vi "testAbbrevDetectorName.vi"(8 "error in (no error)":errorcluster) -> (0 "error out":errorcluster)   [LabVIEW 2016]
doc: "Test to transform the canonical detector name to the abbreviated one."
uses:
  <vilib>/addons/_JKI Toolkits/Caraya/classes/Assert/Assert.lvclass
  <vilib>/addons/_JKI Toolkits/Caraya/classes/Test/Test.lvclass
  MatOper/MatOper.lvclass
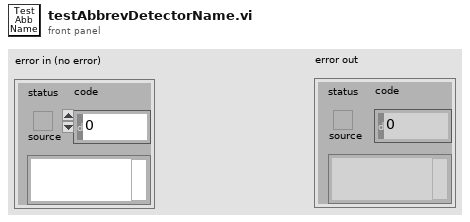
[diagram p1: front panel]
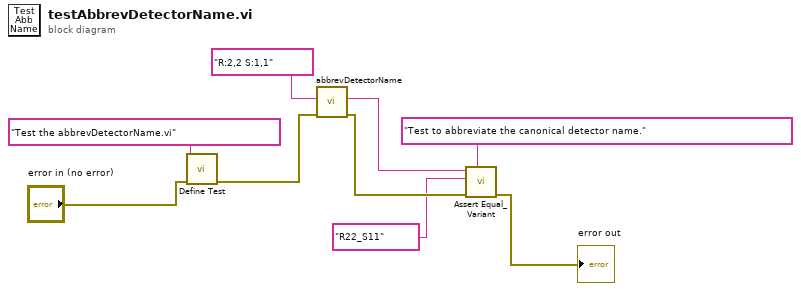
[diagram p0: block diagram]
diagram:
  n1 = call <vilib>:"Define Test.vi"("error in (no error)"="error in (no error)", "Label (VI Title)"="Test the abbrevDetectorName.vi") -> ("error out"=w5:errorcluster)  [unwired: 9 in]
  n2 = call "abbrevDetectorName.vi"("error in (no error)"=w5, "Canonical Name"="R:2,2 S:1,1") -> ("error out"=w4:errorcluster, "Abbreviated Detector Name"=w3:string)  [unwired: 7 in, 1 out]
  n3 = call <vilib>:"Assert Equal_Variant.vi"("Label"="Test to abbreviate the canonical detector name.", "error in (no error)"=w4, "Y"="R22_S11" ("Canonical Name"), "X"=w3) -> ("error out"=→"error out":errorcluster)  [unwired: 7 in]
